vi "Edge detection and search.vi"() -> ()   [LabVIEW 2016]
uses:
  <vilib>/vision/Measure.llb/Edge New.ctl
  <vilib>/userdefined/High Color/IMAQdx.ctl
  <vilib>/vision/driver/NI_Vision_Acquisition_Software.lvlib
  <vilib>/vision/NI_Vision_Development_Module.lvlib
panel:
  in  "Select the Pin to be measured":enum16{"1", "2", "3", "4", "5"}(ring)
  out "Edge Information":T1[](array[typedef]) {"Distance (Real-World)" format="%.2f"; "Location (Real-World)"."Y" format="%.2g"; "Location (Real-World)"."X" format="%.2f"; "Noise" format="%.2f"; "Location (Pixel)"."Y" format="%.2g"; "Location (Pixel)"."X" format="%.2f"; "Strength" format="%.2f"; "Distance (Pixel)" format="%.2f"}
  out "Pixel Column of the edge":sgl
  out "Image":T2(plugin-control)
  in  "File Path":path=path "C:/Users/user/Desktop/Studienarbeit Image Processing/Images Captured/Calibration/Calibration_Target  Grid Distortion_Dot Dia_1mm/Template_Calibrated Image_Exposure_950.png"
  out "error out":errorcluster
  in  "error in (no error)":errorcluster
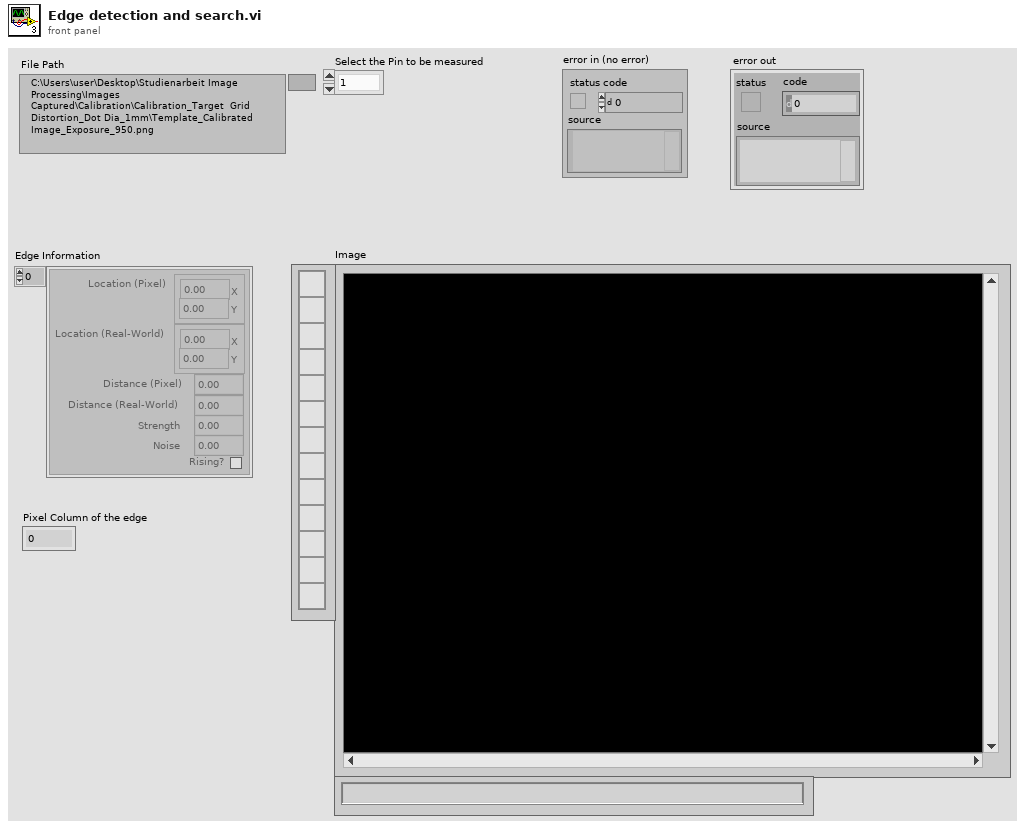
[diagram p1: front panel]
types:
  T1 = typedef "Edge New.ctl" = cluster{"Location (Pixel)":cluster{"X":sgl, "Y":sgl}, "Location (Real-World)":cluster{"X":sgl, "Y":sgl}, "Distance (Pixel)":dbl, "Distance (Real-World)":dbl, "Strength":dbl, "Noise":dbl, "Rising?":bool}
  T2 = typedef "IMAQ Image.ctl" = refnum<image>
  T3 = typedef "IMAQdx.ctl" = refnum<k21>
  T4 = typedef "ROI Descriptor" = cluster{"Global Rectangle":i32[], "Contours":cluster{"ID":enum32{"External", "Internal"}, "Type":u32, "Coordinates":i32[]}[]}
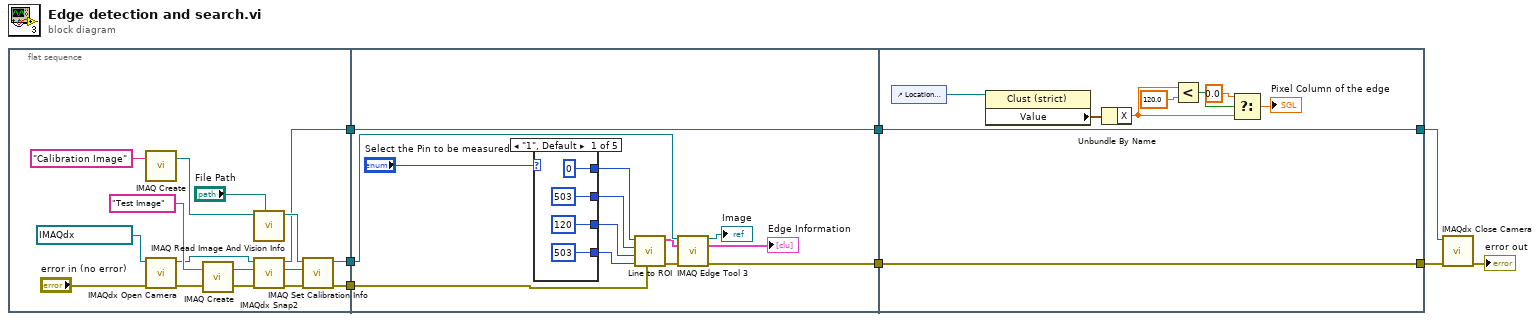
[diagram p0: block diagram]
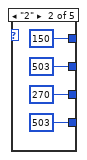
[diagram p2: hidden frame]
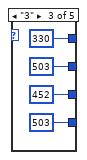
[diagram p3: hidden frame]
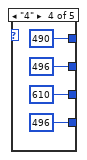
[diagram p4: hidden frame]
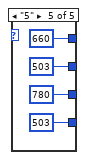
[diagram p5: hidden frame]
diagram:
  n1 = flat-sequence {
    tunnel: [w9] -> w6
    tunnel: [w11] -> w5
    tunnel: [w10] -> w4
    tunnel: w6 -> [w37]
    tunnel: w5 -> [w30]
    tunnel: w4 -> [w35]
    tunnel: [w37] -> w2
    tunnel: [w34] -> w1
    tunnel: [w65] -> w3
    tunnel: [w66] -> w7
    tunnel: w2 -> [w66]
    tunnel: w1 -> [w65]
    frame #0 {
      n2 = call "IMAQ Create"("Image Name"="Calibration Image") -> ("New Image"=w23:T2)  [unwired: 4 in, 1 out]
      n3 = call <vilib>:"IMAQdx Open Camera.vi"("error in"="error in (no error)", "Session In"=T3 "acA780-75gc") -> ("error out"=w17:errorcluster, "Session Out"=w13:T3)  [unwired: 8 in]
      n4 = call "IMAQ Create"("Image Name"="Test Image", "error in (no error)"=w17) -> ("New Image"=w14:T2, "error out"=w18:errorcluster)  [unwired: 3 in]
      n5 = call "IMAQ Read Image And Vision Info"("File Path"="File Path", "Image"=w23) -> ("Image Out"=w21:T2)  [unwired: 7 in, 2 out]
      n6 = call <vilib>:"IMAQdx Snap2.vi"("error in"=w18, "Image In"=w14, "Session In"=w13) -> ("error out"=w19:errorcluster, "Image Out"=w20:T2, "Session Out"=w9:T3)  [unwired: 6 in]
      n7 = call "IMAQ Set Calibration Info"("error in (no error)"=w19, "Image Dst"=w20, "Image Src"=w21) -> ("error out"=w11:errorcluster, "Calibrated Image"=w10:T2)  [unwired: 7 in]
    }
    frame #1 {
      n8 = case shown="\"1\", Default" "Select the Pin to be measured" {
        tunnel: [0 150 ("Start X") 330 ("Start X") 490 ("Start X") 660 ("Start X")] -> w28
        tunnel: [503 503 ("Start X") 503 ("Start X") 496 ("Start X") 503 ("Start X")] -> w27
        tunnel: [120 270 ("Start X") 452 ("Start X") 610 ("Start X") 780 ("Start X")] -> w26
        tunnel: [503 503 ("Start X") 503 ("Start X") 496 ("Start X") 503 ("Start X")] -> w25
        frame "1", Default {
        }
        frame "2" {
        }
        frame "3" {
        }
        frame "4" {
        }
        frame "5" {
        }
      }
      n9 = call "Line to ROI.vi"("error in (no error)"=w30, "End Y"=w25, "End X"=w26, "Start Y"=w27, "Start X"=w28) -> ("error out"=w29:errorcluster, "ROI Descriptor"=w31:T4)  [unwired: 5 in]
      n10 = call "IMAQ Edge Tool 3"("Image"=w35, "ROI Descriptor"=w31, "error in (no error)"=w29) -> ("Image (duplicate)"=→"Image":T2, "Edge Information"=→"Edge Information":T1[], "error out"=w34:errorcluster)  [unwired: 8 in, 2 out]
    }
    frame #2 {
      n11 = control-ref of="Location (Pixel)"() -> (w58:refnum<vi>)
      n12 = property class="Clust (strict)"(reference=w58) -> ("Value"=w59:cluster{"X":sgl, "Y":sgl})  [unwired: 1 in, 2 out]
      n13 = Unbundle By Name(w59) -> ("X"=w63:sgl)
      n14 = Less?(x=w63, y=sgl 120.0) -> (x < y?=w61:bool)
      n15 = Select(t=sgl 0.0, s=w61, f=w63) -> (s? t:f=→"Pixel Column of the edge":sgl)
    }
  }
  n16 = call <vilib>:"IMAQdx Close Camera.vi"("error in"=w3, "Session In"=w7) -> ("error out"=→"error out":errorcluster)  [unwired: 9 in]
